vi "GLdrv_TRANS_SOUR.vi"(0 "Connection ID":T1, 5 "Mode":enum16{"DISK"}(ring), 7 "File Path":string, 11 "error in (no error)":errorcluster, 13 "Query(f)":bool) -> (4 "Connection ID Out":T1, 6 "Mode out":enum16{"DISK"}(ring), 8 "File Path out":string, 15 "error out":errorcluster)   [LabVIEW 2017, in "GL860_Driver.lvlib"]
doc: "データ転送するデータ元を設定・参照します\nDISK：　SDカードを設定します\n例) TRANS:SOUR DISK,”\\SD\\AA.GBD”)\n(詳細はDATAｸﾞﾙｰﾌﾟを参照)"
uses:
  GL860_Driver.lvlib
  ConnectionID.ctl
  GLdrv_RW.ctl
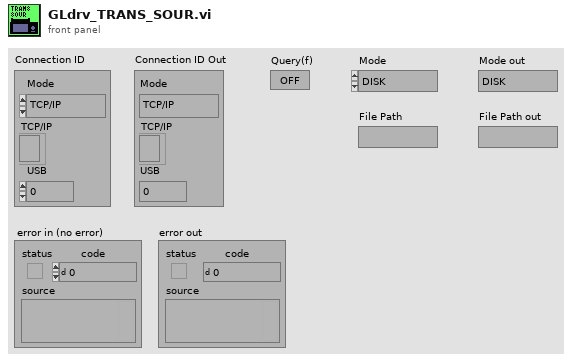
[diagram p1: front panel]
types:
  T1 = typedef "ConnectionID.ctl" = cluster{"Mode":enum16{"TCP/IP", "USB"}, "TCP/IP":refnum<k5>, "USB":i32}
  T2 = typedef "GLdrv_RW.ctl" = enum16{"Auto", "Read", "Write", "Buffer"}
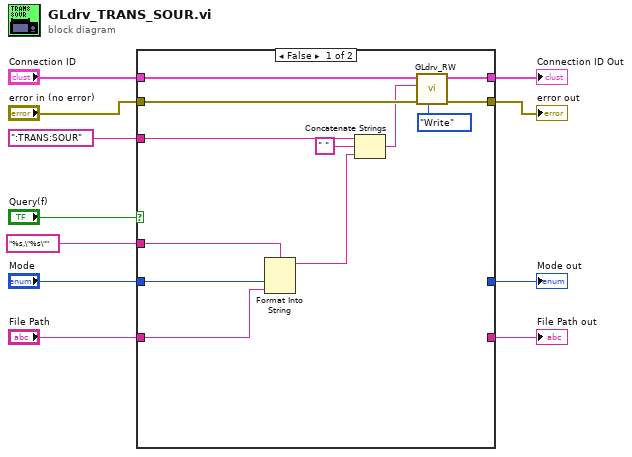
[diagram p0: block diagram]
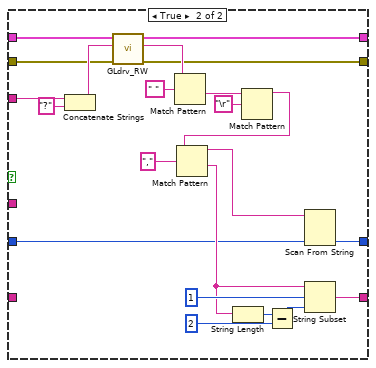
[diagram p2: hidden frame]
diagram:
  n1 = case shown="FALSE" "Query(f)" {
    tunnel: ":TRANS:SOUR" ("Command") -> [w23 w42]
    tunnel: [w18 w35] -> w11
    tunnel: [w20 w39] -> w10
    tunnel: "Connection ID" -> [w21 w40]
    tunnel: "error in (no error)" -> [w19 w36]
    tunnel: "Mode" -> [w14 w24]
    tunnel: [_ w27] -> w3
    tunnel: "%s,\"%s\"" ("Param") -> [w13 _]
    tunnel: "File Path" -> [w12 _]
    tunnel: [_ w26] -> w1
    frame False {
      n2 = Format Into String(format string=w13, w14, w12) -> (resulting string=w15:string)  [unwired: 2 in, 1 out]
      n3 = Concatenate Strings(w23, " " ("string"), w15) -> (w17:string)
      n4 = call "GLdrv_RW.vi"("Mode(read)"=GLdrv_RW."Write", "error in (no error)"=w19, "data in"=w17, "Connection ID"=w21) -> ("error out"=w18:errorcluster, "Connection ID Out"=w20:T1)  [unwired: 3 in, 3 out]
    }
    frame True {
      n5 = Concatenate Strings(w42, "?" ("string")) -> (w38:string)
      n6 = call "GLdrv_RW.vi"("error in (no error)"=w36, "data in"=w38, "Connection ID"=w40) -> ("error out"=w35:errorcluster, "data out"=w37:string, "Connection ID Out"=w39:T1)  [unwired: 4 in, 2 out]
      n7 = Match Pattern(string=w37, regular expression=" " ("search string/char (-)")) -> (after substring=w43:string)  [unwired: 4 out]
      n8 = Match Pattern(string=w43, regular expression="\r") -> (before substring=w25:string)  [unwired: 4 out]
      n9 = Match Pattern(string=w25, regular expression=",") -> (before substring=w33:string, after substring=w28:string)  [unwired: 3 out]
      n10 = String Length(string=w28) -> (length=w31:i32)
      n11 = Subtract(x=w31, y=2) -> (x-y=w30:i32)
      n12 = Scan From String(input string=w33, default 1=w24) -> (output 1=w27:enum16{"DISK"})  [unwired: 3 in, 3 out]
      n13 = String Subset(string=w28, offset (0)=1, length (rest)=w30) -> (substring=w26:string)
    }
  }
  "Connection ID Out" <- w10
  "error out" <- w11
  "Mode out" <- w3
  "File Path out" <- w1
